vi "Offline_Thermal.vi"() -> ()   [LabVIEW 2010]
uses:
  <vilib>/Utility/error.llb/DialogType.ctl
  Types/TYPE Filter Outputs.ctl
  <vilib>/Utility/file.llb/Write To Spreadsheet File (DBL).vi
panel:
  in  "Preamp Gain":dbl(ring)=10.0 items=["10X"=10.0, "100X"=100.0]
  out "Loop Count":i32=84969
  in  "Data File":path=path "C:/Users/Sunderam Lab/Desktop/SEGWAY Labview/NSL11_010716.tdms"
  in  "Temp":bool
  in  "Q Interval":i32=600
  in  "Feature Save To Path":path=path "C:/Users/Sunderam Lab/Desktop/Thermal Code/HMMTest.csv"
  out "Target Temp":dbl=27.0
  out "Temp":dbl=nan
  out "Q":dbl=0.9999999973145681
  out "Temp On":bool
  in  "EEG Coefficients File":path=path "C:/Users/Sunderam Lab/Desktop/Thermal Code/EEG_Coefs.csv"
  in  "Model Information (Mu, Sigma, Priors, Transition Matrix):":path=path "C:/Users/Sunderam Lab/Desktop/SEGWAY Labview/ClusterDataNSL11_010716.csv"
  out "Sleep Stage":i32=2
  out "EEG":waveform(dbl)(graph)={"t0"=timestamp(86400 s since 1904-01-01), "dt"=0.0025, "Y"=[], "attributes"=variant("datatype"=variant(string "DT_DOUBLE"), "description"=variant(string ""), "maximum"=variant(dbl 1366.3837431518552), "minimum"=variant(dbl -1613.23245), "sensitivity"=variant(dbl 1.0))}
  out "EMG":waveform(dbl)(graph)={"t0"=timestamp(86400 s since 1904-01-01), "dt"=0.0025, "Y"=[], "attributes"=variant("datatype"=variant(string "DT_DOUBLE"), "description"=variant(string ""), "maximum"=variant(dbl 1612.592734625244), "minimum"=variant(dbl -1613.23245), "sensitivity"=variant(dbl 1.0))}
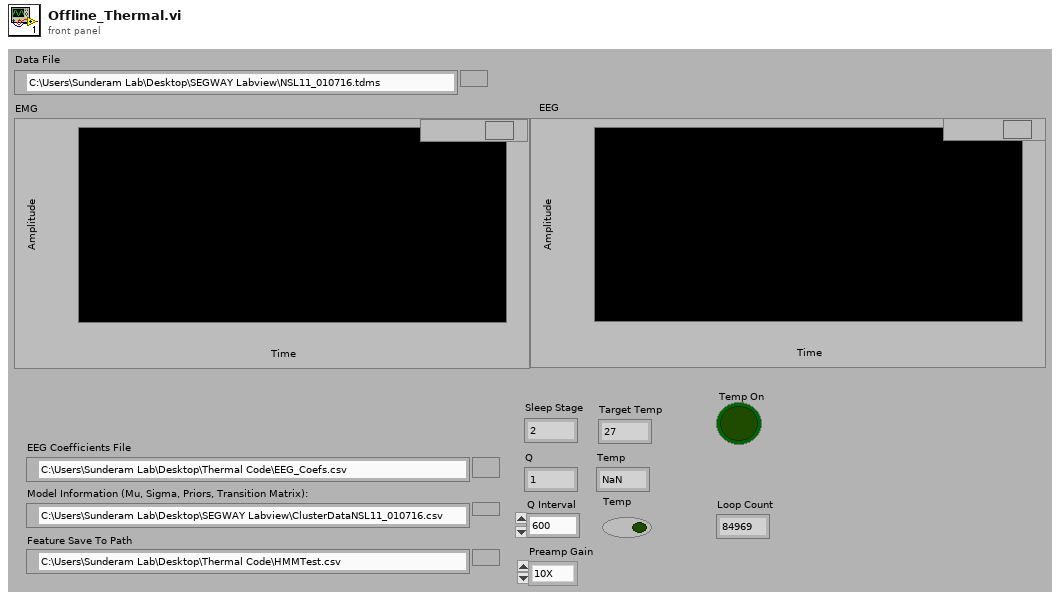
[diagram p1: front panel]
types:
  T1 = typedef "DialogType.ctl" = u16
  T2 = typedef "TYPE Filter Outputs.ctl" = cluster{"Delta:Theta":dbl, "Hi:Lo":dbl, "EMG":dbl, "Delta Low":dbl, "Theta":dbl, "Alpha":dbl, "Beta":dbl, "Gamma":dbl, "Total EEG":dbl, "Detection":dbl, "Stimulate":dbl, "TimeStamp":dbl, "Class Labels":dbl, "Delta High":dbl}
  T3 = typedef "TYPE EEG Components.ctl" = cluster{"Total":dbl, "Alpha":dbl, "Beta":dbl, "Gamma":dbl, "Delta":dbl, "Delta Low":dbl, "Delta High":dbl, "Theta":dbl}
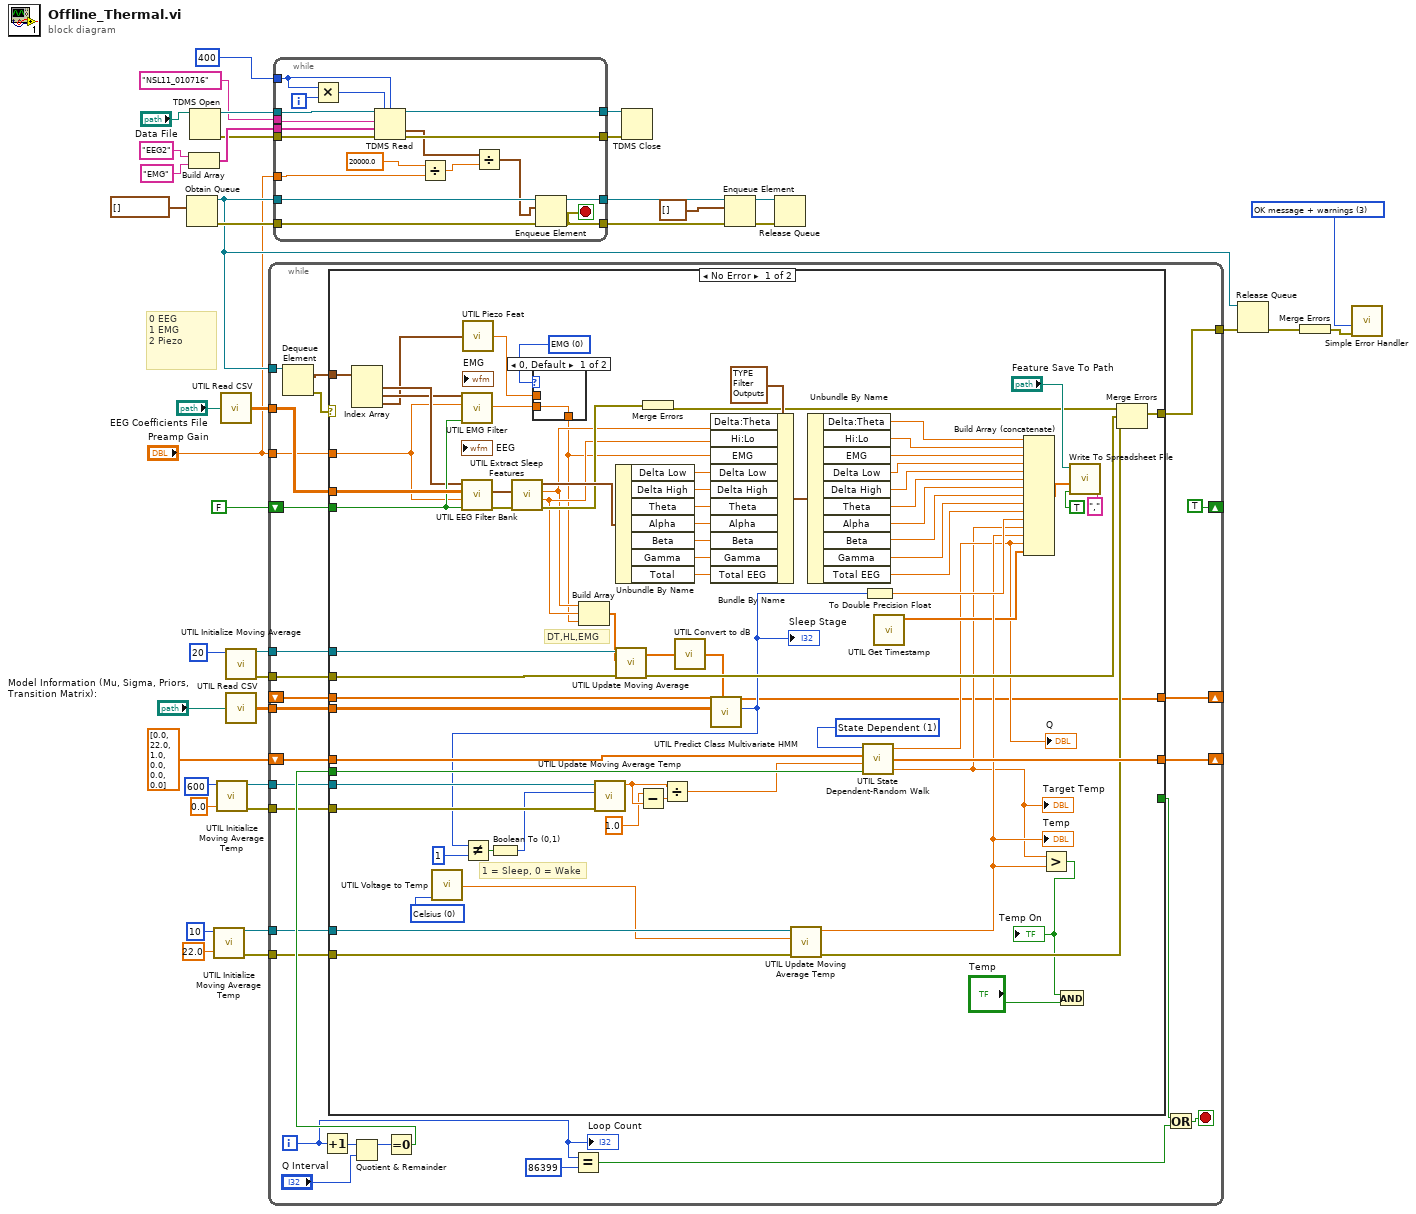
[diagram p0: block diagram]
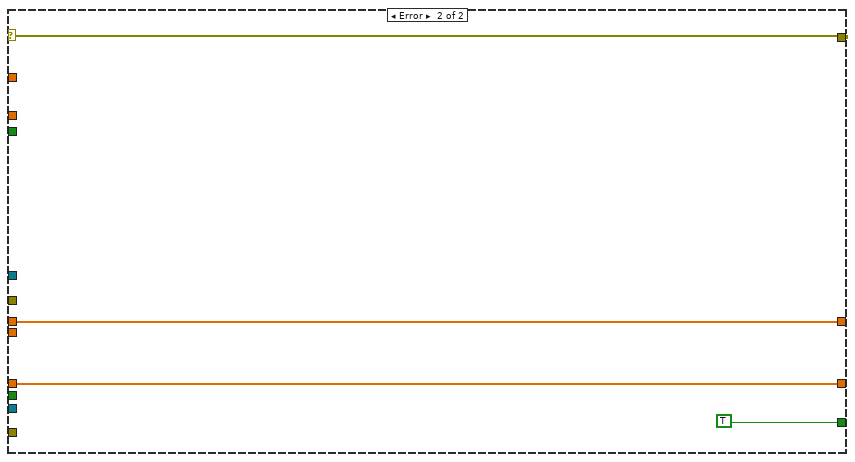
[diagram p3: hidden frame]
diagram:
  w39 = T1 3 items=["no dialog", "OK message", "continue or stop message", "OK message + warnings", "continue/stop + warnings"] ("type of dialog (OK msg:1)")
  # "0 EEG\n1 EMG\n2 Piezo"
  n1 = Obtain Queue(element data type=waveform(dbl)[] [] ("Measurement 2")) -> (queue out=w2:refnum<queue>, error out=w8:errorcluster)  [unwired: 4 in, 1 out]
  n2 = Build Array("EEG2" ("channel name"), "EMG" ("channel name")) -> (w13:string[])
  n3 = TDMS Open(11:"Data File") -> (0:w12:errorcluster, 3:w11:refnum<k34>)  [unwired: 5 in]
  n4 = call "UTIL Initialize Moving Average Temp.vi"("element"=22.0, "Window Width"=10) -> ("Error Out"=w27:errorcluster, "queue out"=w28:refnum<queue>)  [unwired: 8 in]
  n5 = call "UTIL Initialize Moving Average Temp.vi"("element"=0.0, "Window Width"=600) -> ("Error Out"=w24:errorcluster, "queue out"=w25:refnum<queue>)  [unwired: 8 in]
  n6 = call "UTIL Read CSV.vi"("CSV Path"="EEG Coefficients File") -> ("Data From File"=w21:dbl[][])
  n7 = call "UTIL Initialize Moving Average.vi"("Window Width"=20) -> ("Error Out"=w32:errorcluster, "queue out"=w30:refnum<queue>)  [unwired: 9 in]
  n8 = call "UTIL Read CSV.vi"("CSV Path"="Model Information (Mu, Sigma, Priors, Transition Matrix):") -> ("Data From File"=w36:dbl[][])
  n9 = while {
    tunnel: w2 -> [w66]
    shift-right: [TRUE] -> _
    shift-left: FALSE -> [w64]
    tunnel: [w58] -> w38
    tunnel: w32 -> [w61]
    tunnel: w36 -> [w60]
    tunnel: w21 -> [w59]
    shift-right: [w56] -> _
    shift-left: dbl[] [0.0, 22.0, 1.0, 0.0, 0.0, 0.0] ("Parameters Out") -> [w55]
    tunnel: w30 -> [w52]
    tunnel: w28 -> [w51]
    tunnel: w27 -> [w50]
    tunnel: w25 -> [w48]
    tunnel: w24 -> [w47]
    shift-right: [w46] -> _
    shift-left: _ -> [w45]
    tunnel: "Preamp Gain" -> [w41]
    i -> [w44]
    stop <- w63 stop-if-true
    n10 = Dequeue Element(queue=w66) -> (element=w67:waveform(dbl)[], error out=w68:errorcluster)  [unwired: 2 in, 2 out]
    n11 = Increment(x=w44) -> (x+1=w54:i32)
    n12 = Quotient & Remainder(x=w54, y="Q Interval") -> (x-y*floor(x/y)=w57:i32)  [unwired: 1 out]
    n13 = Equal To 0?(x=w57) -> (x = 0?=w53:bool)
    n14 = case shown="No Error" w68 {
      selector: w68 -> [_ w150]
      tunnel: w67 -> [w142 _]
      tunnel: w64 -> [w109 _]
      tunnel: [_ TRUE] -> w62
      tunnel: [w115 w150] -> w58
      tunnel: w61 -> [w108 _]
      tunnel: w60 -> [w126 _]
      tunnel: w59 -> [w111 _]
      tunnel: w53 -> [w114 _]
      tunnel: [w113 w149] -> w56
      tunnel: w55 -> [w99 w149]
      tunnel: w52 -> [w106 _]
      tunnel: w51 -> [w105 _]
      tunnel: w50 -> [w102 _]
      tunnel: w48 -> [w97 _]
      tunnel: w47 -> [w96 _]
      tunnel: [w83 w148] -> w46
      tunnel: w45 -> [w82 w148]
      tunnel: w41 -> [w73 _]
      frame No Error {
        w79 = u16 0 items=["EMG", "Piezo", ""] ("Temperature Units (C)")
        w86 = u16 1 items=["Random Walk", "State Dependent"] ("Temperature Units (C)")
        w112 = u16 0 items=["Celsius", "Fahrenheit", "Kelvin", "Rankine"] ("Temperature Units (C)")
        # "1 = Sleep, 0 = Wake"
        # "DT,HL,EMG"
        n15 = Index Array(array=w142) -> (element #1=w78:waveform(dbl), element #2=w77:waveform(dbl), element #3=w72:waveform(dbl))  [unwired: 3 in]
        n16 = call "UTIL Voltage to Temp.vi"("Temperature Units (C)"=w112) -> ("Temp"=w104:dbl)  [unwired: 10 in]
        n17 = call "UTIL EMG Filter.vi"("init/cont (init:F)"=w109, "Preamp Gain"=w73, "EMG In"=w77) -> ("EMG Power"=w81:dbl)  [unwired: 7 in, 1 out]
        n18 = call "UTIL EEG Filter Bank.vi"("init/cont (init:F)"=w109, "Amplifier Gain"=w73, "Filter Coefficients from File"=w111, "EEG In"=w78) -> ("Error Out"=w145:errorcluster, "EEG Components"=w110:T3)  [unwired: 5 in, 1 out]
        n19 = call "UTIL Piezo Feat.vi"("Piezo In"=w72) -> ("Piezo Power"=w80:dbl)  [unwired: 4 in]
        n20 = call "UTIL Extract Sleep Features.vi"("Error In"=w145, "Components In"=w110) -> ("Error Out"=w127:errorcluster, "Hi:Lo"=w76:dbl, "Delta:Theta"=w75:dbl, "Components Out"=w143:T3)  [unwired: 6 in]
        n21 = case shown="0, Default" w79 {
          tunnel: w81 -> [w146 _]
          tunnel: w80 -> [_ w147]
          tunnel: [w146 w147] -> w74
          frame 0, Default {
          }
          frame 1 {
          }
        }
        n22 = Build Array(w75, w76, w74) -> (w71:dbl[])
        n23 = Unbundle By Name(w143) -> ("Delta Low"=w125:dbl, "Delta High"=w124:dbl, "Theta"=w123:dbl, "Alpha"=w122:dbl, "Beta"=w121:dbl, "Gamma"=w120:dbl, "Total"=w119:dbl)
        n24 = call "UTIL Update Moving Average.vi"("Error In"=w108, "Data In"=w71, "Average Queue"=w106) -> ("Error Out"=w107:errorcluster, "Average"=w70:dbl[])  [unwired: 7 in]
        n25 = Merge Errors(w127) -> (w116:errorcluster)
        n26 = call "UTIL Convert to dB.vi"("Features In"=w70) -> ("Features (dB)"=w69:dbl[])
        n27 = Bundle By Name(cluster=T2 {"Delta:Theta"=0.0, "Hi:Lo"=0.0, "EMG"=0.0, "Delta Low"=0.0, "Theta"=0.0, "Alpha"=0.0, "Beta"=0.0, "Gamma"=0.0, "Total EEG"=0.0, "Detection"=0.0, "Stimulate"=0.0, "TimeStamp"=0.0, "Class Labels"=0.0, "Delta High"=0.0} ("Filter Outputs"), "Delta:Theta"=w75, "Hi:Lo"=w76, "EMG"=w74, "Delta Low"=w125, "Delta High"=w124, "Theta"=w123, "Alpha"=w122, "Beta"=w121, "Gamma"=w120, "Total EEG"=w119) -> (w141:T2)
        n28 = call "UTIL Predict Class Multivariate HMM.vi"("Data Point"=w69, "Model Information"=w126, "d(t-1) In"=w82) -> ("Sleep Stage"=w84:i32, "d(t-1) Out"=w83:dbl[])  [unwired: 5 in]
        "Sleep Stage" <- w84
        n29 = Not Equal?(x=w84, y=1) -> (x != y?=w94:bool)
        n30 = Boolean To (0,1)(Boolean=w94) -> (0, 1=w93:i16)
        n31 = call "UTIL Update Moving Average Temp.vi"("Error In"=w96, "Data Point"=w93, "Average Queue"=w97) -> ("Moving Average"=w91:dbl)  [unwired: 7 in, 1 out]
        n32 = Subtract(x=1.0, y=w91) -> (x-y=w92:dbl)
        n33 = Divide(x=w91, y=w92) -> (x/y=w89:dbl)
        n34 = call "UTIL Update Moving Average Temp.vi"("Error In"=w102, "Data Point"=w104, "Average Queue"=w105) -> ("Error Out"=w101:errorcluster, "Moving Average"=w103:dbl)  [unwired: 7 in]
        "Temp" <- w103
        n35 = Unbundle By Name(w141) -> ("Delta:Theta"=w140:dbl, "Hi:Lo"=w139:dbl, "EMG"=w138:dbl, "Delta Low"=w137:dbl, "Delta High"=w129:dbl, "Theta"=w130:dbl, "Alpha"=w131:dbl, "Beta"=w132:dbl, "Gamma"=w136:dbl, "Total EEG"=w118:dbl)
        n36 = call "UTIL State Dependent-Random Walk.vi"("Boolean"=w114, "Numeric"=w89, "Parameters Out"=w99, "Temperature Units (C)"=w86) -> ("Target Temp"=w85:dbl, "Parameters Out"=w113:dbl[], "Q"=w98:dbl)
        "Q" <- w98
        "Target Temp" <- w85
        n37 = To Double Precision Float(number=w84) -> (double precision float=w117:dbl)
        n38 = call "UTIL Get Timestamp.vi"() -> ("appended array"=w100:dbl[])  [unwired: 7 in, 1 out]
        n39 = Build Array (concatenate)(w140, w139, w138, w137, w129, w130, w131, w132, w136, w118, w117, w85, w103, w98, w100) -> (w128:dbl[])
        n40 = Greater?(x=w85, y=w103) -> (0:w87:bool)
        "Temp On" <- w87
        n41 = And(x=w87, y="Temp") -> ()  [unwired: 1 out]
        n42 = call-poly <vilib>:"Write To Spreadsheet File.vi"("delimiter (\\t)"="," ("delimiter (\\t)"), "append to file? (new file:F)"=TRUE, "1D data"=w128, "file path (dialog if empty)"="Feature Save To Path") -> ()  [unwired: 4 in, 1 out]
        n43 = Merge Errors(w116, w107, w101) -> (w115:errorcluster)
      }
      frame Error {
      }
    }
    n44 = Equal?(x=w44, y=86399) -> (x = y?=w42:bool)
    n45 = Or(x=w62, y=w42) -> (x .or. y?=w63:bool)
    "Loop Count" <- w44
  }
  n46 = while {
    tunnel: w11 -> [w165]
    tunnel: w12 -> [w167]
    tunnel: 400 -> [w169]
    tunnel: [w168] -> w19
    tunnel: [w166] -> w17
    tunnel: w13 -> [w164]
    tunnel: "NSL11_010716" ("group name") -> [w163]
    tunnel: w2 -> [w161]
    tunnel: w8 -> [w160]
    tunnel: [w159] -> w7
    tunnel: [w158] -> w6
    tunnel: "Preamp Gain" -> [w152]
    i -> [w162]
    stop <- w158 stop-if-true
    n47 = Multiply(x=w169, y=w162) -> (x*y=w157:i32)
    n48 = TDMS Read(0:w165, 1:w157, 2:w169, 5:w163, 7:w164, 11:w167) -> (4:w166:refnum<k34>, 10:w156:waveform(dbl)[], 15:w168:errorcluster)  [unwired: 1 in, 3 out]
    n49 = Divide(x=20000.0 ("y"), y=w152) -> (x/y=w154:dbl)
    n50 = Divide(x=w156, y=w154) -> (x/y=w155:waveform(dbl)[])
    n51 = Enqueue Element(queue=w161, element=w155, error in (no error)=w160) -> (queue out=w159:refnum<queue>, error out=w158:errorcluster)  [unwired: 1 in, 1 out]
  }
  n52 = TDMS Close(8:w19, 11:w17) -> ()  [unwired: 2 out]
  n53 = Enqueue Element(queue=w7, element=waveform(dbl)[] [] ("Measurement 2"), error in (no error)=w6) -> (queue out=w4:refnum<queue>, error out=w3:errorcluster)  [unwired: 1 in, 1 out]
  n54 = Release Queue(queue=w4, error in (no error)=w3) -> ()  [unwired: 1 in, 3 out]
  n55 = Release Queue(queue=w2, error in (no error)=w38) -> (error out=w33:errorcluster)  [unwired: 1 in, 2 out]
  n56 = Merge Errors(w33) -> (w34:errorcluster)
  n57 = call <vilib>:"Simple Error Handler.vi"("type of dialog (OK msg:1)"=w39, "error in (no error)"=w34) -> ()  [unwired: 3 in, 5 out]
